vi "test Get and Set State.vi"(8 "error in (no error)":errorcluster, 11 "TestCase in":refnum<class "Framework Property Tests.lvclass">) -> (0 "error out":errorcluster, 3 "TestCase out":refnum<class "Framework Property Tests.lvclass">)   [LabVIEW 2017, in "Framework Property Tests.lvclass"]
uses:
  Framework Property Tests.lvclass
  Engine/Classes/Framework/Framework.lvclass
  Engine/Classes/State/Framework State.lvclass
  Engine/Classes/State/Framework State.lvclass/Framework State.ctl
  Engine/Classes/Framework/Framework.lvclass/Framework.ctl
  <vilib>/addons/_JKI Toolkits/VI Tester/TestCase.llb/TestCase.lvclass
  C:/Program Files (x86)/National Instruments/LabVIEW 2017/vi.lib/addons/_JKI Toolkits/VI Tester/TestCase.llb/TestCase.lvclass
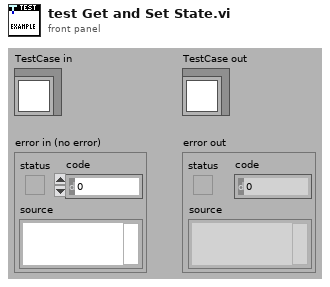
[diagram p1: front panel]
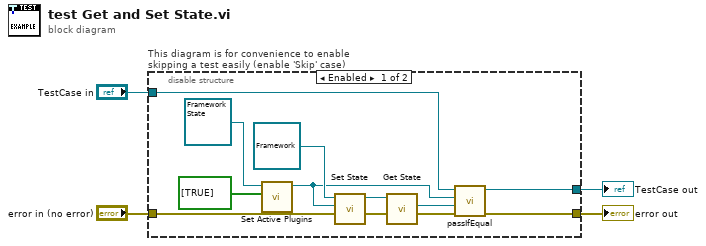
[diagram p0: block diagram]
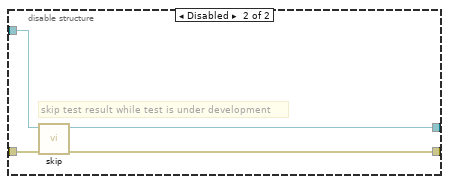
[diagram p2: hidden frame]
diagram:
  n1 = disable-structure "This diagram is for convenience to enable skipping a test easily (enable 'Skip' case)" shown="Enabled" {
    disable-tunnel: "TestCase in" -> [w11 w18]
    disable-tunnel: [w10 w16] -> w2
    disable-tunnel: [w12 w17] -> w1
    disable-tunnel: "error in (no error)" -> [w14 w15]
    frame Enabled {
      n2 = call "Set Active Plugins.vi"("Active Plugins"=bool[] [TRUE], "Framework State in"=refnum<class "Framework State.lvclass"> refnum ("State")) -> ("Framework State out"=w6:refnum<class "Framework State.lvclass">)  [unwired: 9 in]
      n3 = call "Set State.vi"("State"=w6, "Framework in"=refnum<class "Framework.lvclass"> refnum ("Mock Framework in")) -> ("Framework out"=w9:refnum<class "Framework.lvclass">)  [unwired: 9 in]
      n4 = call "Get State.vi"("Framework in"=w9) -> ("State"=w8:refnum<class "Framework State.lvclass">)  [unwired: 9 in, 1 out]
      n5 = call-dynamic "passIfEqual.vi"("error in (no error)"=w14, "y"=w8, "x"=w6, "TestCase in"=w11) -> ("error out"=w12:errorcluster, "TestCase out"=w10:refnum<class "Framework Property Tests.lvclass">)  [unwired: 6 in]
    }
    frame Disabled {
      # "skip test result while test is under development"
      n6 = call <vilib>:"skip.vi"("error in (no error)"=w15, "TestCase in"=w18) -> ("error out"=w17:errorcluster, "TestCase out"=w16:refnum<class "Framework Property Tests.lvclass">)  [unwired: 8 in]
    }
  }
  "error out" <- w1
  "TestCase out" <- w2
